vi "ma_FFT with Hanning (CDB).vi"(11 "time signal data":cdb[](array[numeric])) -> (2 "FFT size":i32, 3 "complex Hann spectrum":cdb[](array[numeric]))   [LabVIEW 2020, in "NI_MAPro.lvlib"]
uses:
  NI_MAPro.lvlib
  AllCosWindow (CDB).vi
  NI_AALPro.lvlib
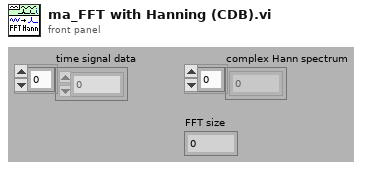
[diagram p1: front panel]
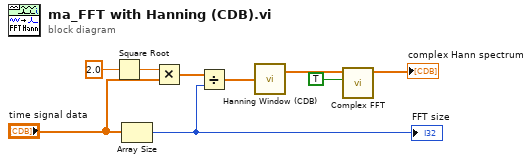
[diagram p0: block diagram]
diagram:
  n1 = Square Root(x=2.0) -> (sqrt(x)=w8:dbl)
  n2 = Array Size(array="time signal data") -> (size(s)=w1:i32)
  "FFT size" <- w1
  n3 = Multiply(x=w8, y="time signal data") -> (x*y=w9:cdb[])
  n4 = Divide(x=w9, y=w1) -> (x/y=w4:cdb[])
  n5 = call "Hanning Window (CDB).vi"("X"=w4) -> ("Windowed X"=w6:cdb[])  [unwired: 1 out]
  n6 = call "Complex FFT.vi"("shift?"=TRUE, "X"=w6) -> ("FFT {X}"=→"complex Hann spectrum":cdb[])  [unwired: 8 in, 1 out]
